vi "PH_Beckhoff.evt Call Set Double Value.vi"(0 "i ref in":refnum<vi>, 2 "Beckhoff Instance":string, 3 "Tagname to set":string, 4 "Value":dbl, 5 "error in":errorcluster) -> (14 "i ref out":refnum<vi>, 19 "error out":errorcluster)   [LabVIEW 2014, in "PH_Beckhoff.lvlib"]
uses:
  PH_Beckhoff.lvlib
  CSCore/CSSystem/CoreLib/CoreLib.string 2 byte array.vi
  CSCore/CSSystem/CoreLib/CoreLib.double 2 byte array.vi
  CSCore/BaseProcess/BaseProcess.lvlib
  CSCore/CSSystem/CoreLib/CoreLib.lvlib
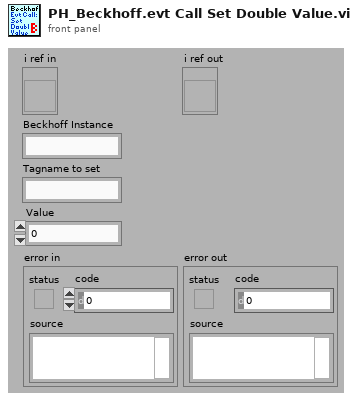
[diagram p1: front panel]
types:
  T1 = typedef "CoreDefs.rawDataType.ctl" = i8[]
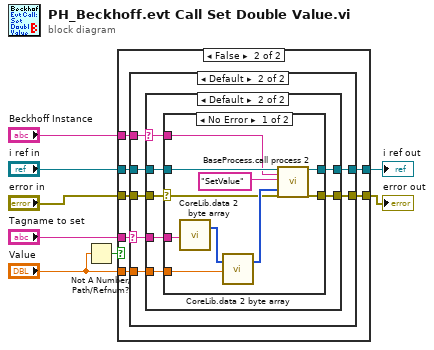
[diagram p0: block diagram]
diagram:
  n1 = Not A Number/Path/Refnum?(number/path/refnum="Value") -> (NaN/Path/Refnum?=w2:bool)
  n2 = case shown="False" w2 {
    tunnel: "error in" -> [w9 w17]
    tunnel: "Value" -> [_ w16]
    tunnel: [w10 w15] -> w7
    tunnel: "i ref in" -> [w10 w14]
    tunnel: [w9 w13] -> w5
    tunnel: "Beckhoff Instance" -> [_ w12]
    tunnel: "Tagname to set" -> [_ w11]
    frame True {
    }
    frame False {
      n3 = case shown="Default" w11 {
        selector: w11 -> [_ w20]
        tunnel: w17 -> [w18 w26]
        tunnel: w16 -> [_ w25]
        tunnel: [w19 w24] -> w15
        tunnel: w14 -> [w19 w23]
        tunnel: [w18 w22] -> w13
        tunnel: w12 -> [_ w21]
        frame "", "N/A" {
        }
        frame Default {
          n4 = case shown="Default" w21 {
            selector: w21 -> [_ w29]
            tunnel: w26 -> [w27 w35]
            tunnel: w25 -> [_ w34]
            tunnel: w20 -> [_ w33]
            tunnel: [w28 w32] -> w24
            tunnel: w23 -> [w28 w31]
            tunnel: [w27 w30] -> w22
            frame "", "N/A" {
            }
            frame Default {
              n5 = case shown="No Error" w35 {
                selector: w35 -> [w37 w46]
                tunnel: [w45 w46] -> w30
                tunnel: w31 -> [w44 w47]
                tunnel: [w43 w47] -> w32
                tunnel: w29 -> [w42 _]
                tunnel: w33 -> [w38 _]
                tunnel: w34 -> [w36 _]
                frame No Error {
                  n6 = call-poly "CoreLib.data 2 byte array.vi"("string"=w38) -> ("byteArray out"=w40:T1)  [unwired: 18 in]
                  n7 = call-poly "CoreLib.data 2 byte array.vi"("byteArray"=w40, "f64"=w36) -> ("byteArray out"=w39:T1)  [unwired: 17 in]
                  n8 = call "BaseProcess.call process 2.vi"("i ref in"=w44, "Object"=w42, "Selector"="SetValue", "Data"=w39, "error in (no error)"=w37) -> ("i ref out"=w43:refnum<vi>, "error out"=w45:errorcluster)  [unwired: 13 in]
                }
                frame Error {
                }
              }
            }
          }
        }
      }
    }
  }
  "i ref out" <- w7
  "error out" <- w5
